vi "Connect.vi"(8 "error in (no error)":errorcluster, 11 "Modeli in":refnum<class "Modeli.lvclass">) -> (0 "error out":errorcluster, 2 "Event Registration Refnum":refnum<event-registration>, 3 "Modeli out":refnum<class "Modeli.lvclass">)   [LabVIEW 2018, in "Modeli.lvlib" / "Modeli.lvclass"]
uses:
  Modeli.lvclass
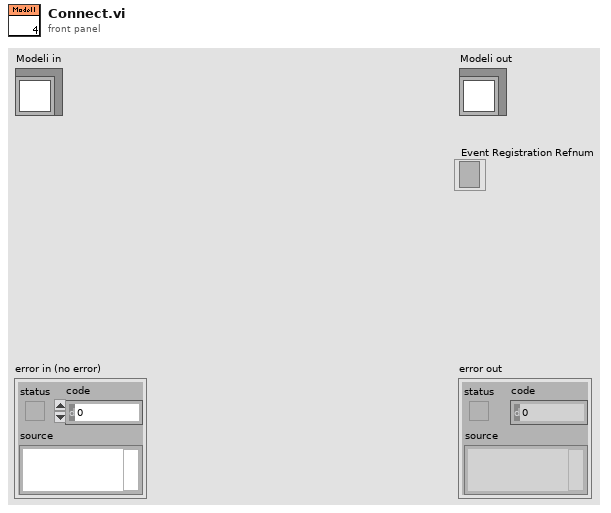
[diagram p1: front panel]
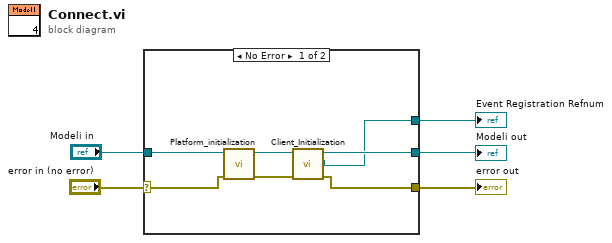
[diagram p0: block diagram]
diagram:
  n1 = case shown="No Error" "error in (no error)" {
    selector: "error in (no error)" -> [w9 w13]
    tunnel: "Modeli in" -> [w12 w14]
    tunnel: [w10 w14] -> w3
    tunnel: [w7 w13] -> w2
    tunnel: [w6 _] -> w1
    frame No Error {
      n2 = call "Platform_initialization.vi"("error in (no error)"=w9, "Modeli in"=w12) -> ("error out"=w8:errorcluster, "Modeli out"=w11:refnum<class "Modeli.lvclass">)  [unwired: 8 in]
      n3 = call "Client_Initialization.vi"("error in (no error)"=w8, "Modeli.lvlib:Modeli.lvclass"=w11) -> ("error out"=w7:errorcluster, "Event Registration Refnum"=w6:refnum<event-registration>, "Modeli.lvlib:Modeli.lvclass 2"=w10:refnum<class "Modeli.lvclass">)  [unwired: 7 in]
    }
    frame Error {
    }
  }
  "error out" <- w2
  "Modeli out" <- w3
  "Event Registration Refnum" <- w1
